vi "Read Key Value - Path.vi"(4 "Default":path, 7 "application directory":path, 8 "error in (no error)":errorcluster, 9 "key":string, 10 "section":string, 11 "file refnum in":T1) -> (0 "error out":errorcluster, 2 "value":path, 3 "file refnum out":T1)   [LabVIEW 2019, in "TSC File IO.lvlib"]
doc: "This VI will read a section/key configuration file and return:\n<b>Path</b>\n\n<b>Note:</b> The VI will resolve relative paths that will be relative to the input ini file path and the symbolic paths. This gives flexibility to defining key/value pairs for absolute and relative paths.\n\n<appdir> : use the input application directory or the application directory primative (if blank)\n<temp> : the OS temporary directory\n<userdoc> : logged in user's documents folder (Windows)\n<userdesktop> : logged in user's desktop folder (Windows)\n<programdata> : ProgramData folder (Windows)\n<bootdir> : the OS install drive (Windows)\n<programfiles> : the installation directory of applications (Windows)\n..\\ : nomenclature of relative path to the ini file directory\n\nInputs:\n-file refnum in [ref] - the reference to the open config file\n-section [string] - the section string in the configuration file\n-key [string] - the key to be read in the configuration file\n-error in\n\nOutputs:\n-file refnum out [ref] - the reference to the open config file\n-value [Path] - the output data read\n-error out\n\n<b>Code Developed By:</b>\nDaniel Coons\nTechnology Service Corporation\n1983 S Liberty Drive\nBloomington, IN 47403\nwww.tsc.com\\atcs"
uses:
  TSC File IO.lvlib
  <vilib>/Utility/config.llb/Config Data RefNum.ctl
  <vilib>/Utility/sysdir.llb/System Directory Type.ctl
  <vilib>/Utility/config.llb/Read Key (Path).vi
  <vilib>/Utility/config.llb/NI_LVConfig.lvlib
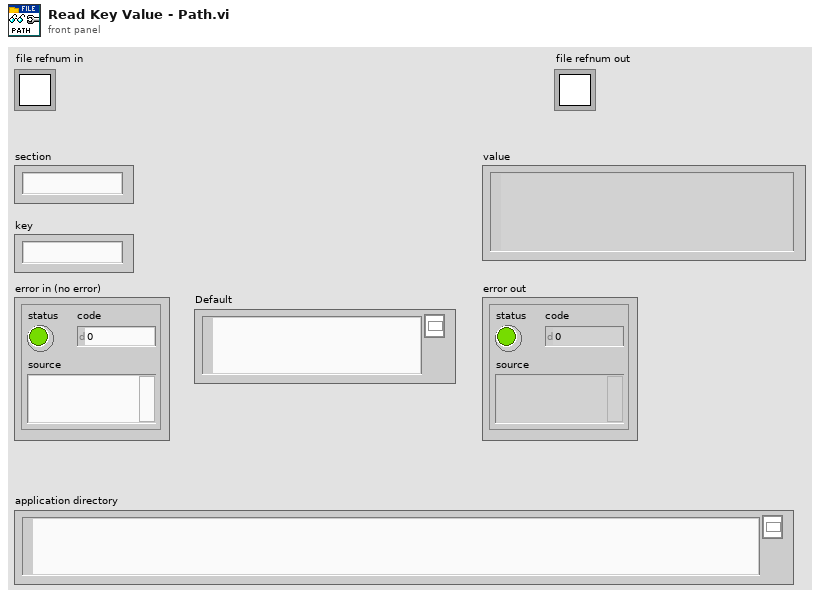
[diagram p1: front panel]
types:
  T1 = typedef "NI_LVConfig.lvlib/Config Data RefNum.ctl" = refnum<k1>
  T2 = typedef "System Directory Type.ctl" = i32
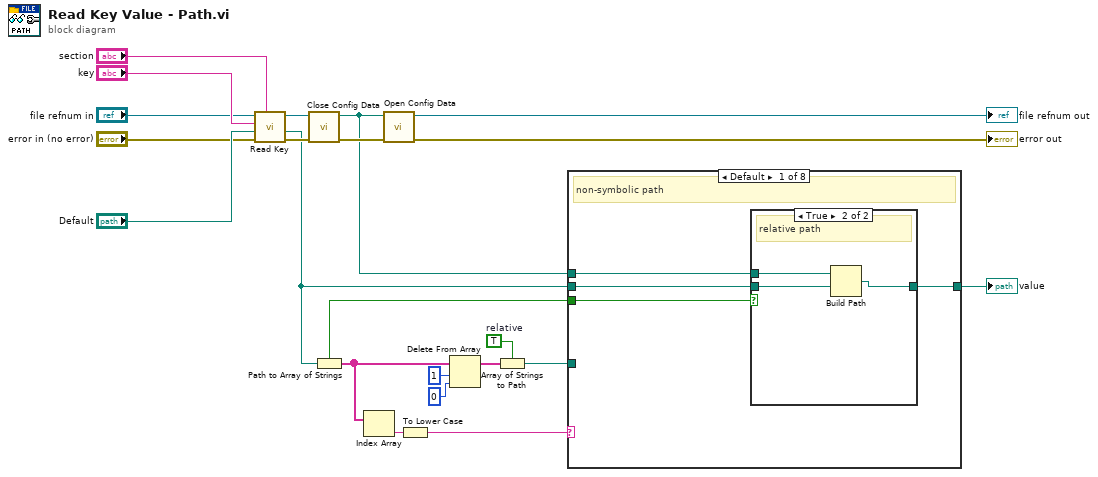
[diagram p0: block diagram]
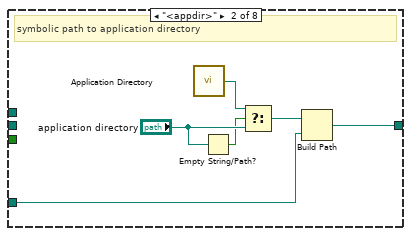
[diagram p3: hidden frame]
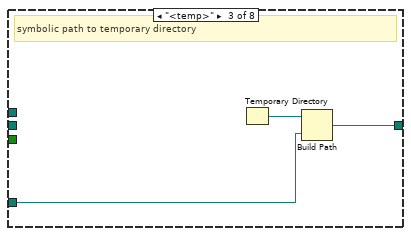
[diagram p4: hidden frame]
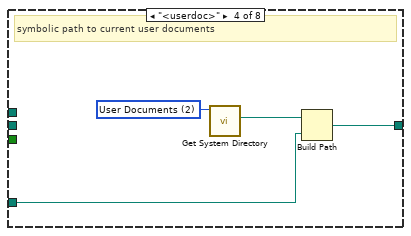
[diagram p5: hidden frame]
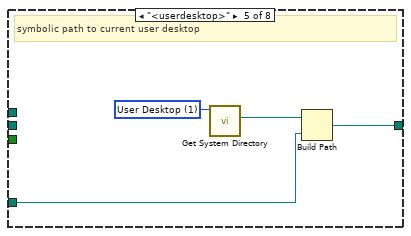
[diagram p6: hidden frame]
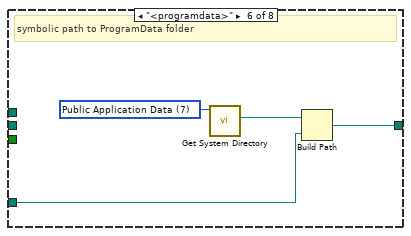
[diagram p7: hidden frame]
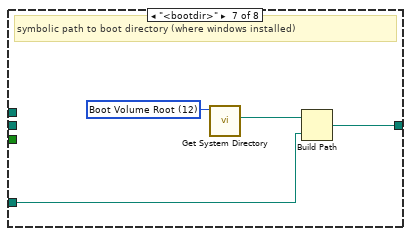
[diagram p8: hidden frame]
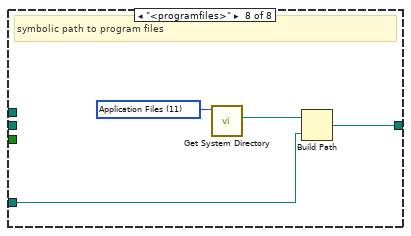
[diagram p9: hidden frame]
diagram:
  w10 = TRUE  # relative
  n1 = call-poly <vilib>:"Read Key.vi"("section"="section", "error in (no error)"="error in (no error)", "default value"="Default", "key"="key", "refnum"="file refnum in") -> ("error out"=w19:errorcluster, "value"=w16:path, "refnum out"=w20:T1)  [unwired: 3 in, 1 out]
  n2 = call <vilib>:"Close Config Data.vi"("error in (no error)"=w19, "refnum"=w20) -> ("error out"=w13:errorcluster, "file path"=w2:path)  [unwired: 8 in]
  n3 = Path to Array of Strings(0:w16) -> (1:w15:bool, 2:w6:string[])
  n4 = Index Array(array=w6) -> (element=w17:string)  [unwired: 1 in]
  n5 = call <vilib>:"Open Config Data.vi"("error in (no error)"=w13, "configuration file path"=w2) -> ("error out"=→"error out":errorcluster, "refnum"=→"file refnum out":T1)  [unwired: 7 in, 1 out]
  n6 = To Lower Case(string=w17) -> (all lower case string=w12:string)
  n7 = Delete From Array(array=w6, length=1, index=0) -> (array with subset deleted=w11:string[])  [unwired: 1 out]
  n8 = Array of Strings to Path(0:w11, 1:w10) -> (2:w7:path)
  n9 = case shown="Default" w12 {
    tunnel: w16 -> [w25 _ _ _ _ _ _ _]
    tunnel: w15 -> [w26 _ _ _ _ _ _ _]
    tunnel: [w24 w36 w39 w43 w47 w51 w55 w59] -> w14
    tunnel: w2 -> [w23 _ _ _ _ _ _ _]
    tunnel: w7 -> [_ w31 w37 w42 w46 w50 w54 w58]
    frame Default {
      # "non-symbolic path"
      n10 = case shown="True" w26 {
        tunnel: w25 -> [w27 w28]
        tunnel: [w27 w29] -> w24
        tunnel: w23 -> [_ w30]
        frame False {
          # "absolute path"
        }
        frame True {
          # "relative path"
          n11 = Build Path(base path=w30, name or relative path=w28) -> (appended path=w29:path)
        }
      }
    }
    frame "<appdir>" {
      # "symbolic path to application directory"
      n12 = call <vilib>:"Application Directory.vi"() -> ("Application Directory"=w35:path)
      n13 = Empty String/Path?(string/path="application directory") -> (empty?=w33:bool)
      n14 = Select(t=w35, s=w33, f="application directory") -> (s? t:f=w32:path)
      n15 = Build Path(base path=w32, name or relative path=w31) -> (appended path=w36:path)
    }
    frame "<temp>" {
      # "symbolic path to temporary directory"
      n16 = Temporary Directory() -> (w38:path)
      n17 = Build Path(base path=w38, name or relative path=w37) -> (appended path=w39:path)
    }
    frame "<userdoc>" {
      w41 = T2 2 items=["User Home"=0, "User Desktop"=1, "User Documents"=2, "User Application Data"=3, "User Preferences"=4, "User Temporary"=5, "Public Documents"=6, "Public Application Data"=7, "Public Preferences"=8, "Public Cache"=13, "System Core Libraries"=9, "System Installed Libraries"=10, "Application Files"=11, "Boot Volume Root"=12] ("system directory type")
      # "symbolic path to current user documents"
      n18 = call <vilib>:"Get System Directory.vi"("system directory type"=w41) -> ("system directory"=w40:path)  [unwired: 10 in]
      n19 = Build Path(base path=w40, name or relative path=w42) -> (appended path=w43:path)
    }
    frame "<userdesktop>" {
      w45 = T2 1 items=["User Home"=0, "User Desktop"=1, "User Documents"=2, "User Application Data"=3, "User Preferences"=4, "User Temporary"=5, "Public Documents"=6, "Public Application Data"=7, "Public Preferences"=8, "Public Cache"=13, "System Core Libraries"=9, "System Installed Libraries"=10, "Application Files"=11, "Boot Volume Root"=12] ("system directory type")
      # "symbolic path to current user desktop"
      n20 = call <vilib>:"Get System Directory.vi"("system directory type"=w45) -> ("system directory"=w44:path)  [unwired: 10 in]
      n21 = Build Path(base path=w44, name or relative path=w46) -> (appended path=w47:path)
    }
    frame "<programdata>" {
      w49 = T2 7 items=["User Home"=0, "User Desktop"=1, "User Documents"=2, "User Application Data"=3, "User Preferences"=4, "User Temporary"=5, "Public Documents"=6, "Public Application Data"=7, "Public Preferences"=8, "Public Cache"=13, "System Core Libraries"=9, "System Installed Libraries"=10, "Application Files"=11, "Boot Volume Root"=12] ("system directory type")
      # "symbolic path to ProgramData folder"
      n22 = call <vilib>:"Get System Directory.vi"("system directory type"=w49) -> ("system directory"=w48:path)  [unwired: 10 in]
      n23 = Build Path(base path=w48, name or relative path=w50) -> (appended path=w51:path)
    }
    frame "<bootdir>" {
      w53 = T2 12 items=["User Home"=0, "User Desktop"=1, "User Documents"=2, "User Application Data"=3, "User Preferences"=4, "User Temporary"=5, "Public Documents"=6, "Public Application Data"=7, "Public Preferences"=8, "Public Cache"=13, "System Core Libraries"=9, "System Installed Libraries"=10, "Application Files"=11, "Boot Volume Root"=12] ("system directory type")
      # "symbolic path to boot directory (where windows installed)"
      n24 = call <vilib>:"Get System Directory.vi"("system directory type"=w53) -> ("system directory"=w52:path)  [unwired: 10 in]
      n25 = Build Path(base path=w52, name or relative path=w54) -> (appended path=w55:path)
    }
    frame "<programfiles>" {
      w57 = T2 11 items=["User Home"=0, "User Desktop"=1, "User Documents"=2, "User Application Data"=3, "User Preferences"=4, "User Temporary"=5, "Public Documents"=6, "Public Application Data"=7, "Public Preferences"=8, "Public Cache"=13, "System Core Libraries"=9, "System Installed Libraries"=10, "Application Files"=11, "Boot Volume Root"=12] ("system directory type")
      # "symbolic path to program files"
      n26 = call <vilib>:"Get System Directory.vi"("system directory type"=w57) -> ("system directory"=w56:path)  [unwired: 10 in]
      n27 = Build Path(base path=w56, name or relative path=w58) -> (appended path=w59:path)
    }
  }
  "value" <- w14
